vi "Console with Filter.vi"() -> ()   [LabVIEW 2019]
uses:
  Log/Log.lvclass
  Log Sinks/Sink-Console/Sink-Console.lvclass
  Log/Event Level.ctl
  TSC Event Logger.lvlib
  Layouts/SimpleLayout/SimpleLayout.lvclass
  Layouts/CSVLayout/CSVLayout.lvclass
  Layouts/JSONLayout/JSONLayout.lvclass
  Log Sinks/Sink-Console/Construct - Input.vi
  e05bdbe4-a397-4cd1-a311-50e4536787bd.vi
  C:/Development/Reuse-libraries/Event Logger/Layouts/Layout.lvclass
  C:/Development/Reuse-libraries/Event Logger/Log Sinks/Log Sinks.lvclass
panel:
  out "string array":string[][](array[string])
  in  "Level Filter":T1=enum."INFO"
  in  "Event Filter":string
  in  "Source Filter":string
  in  "Layout":enum16{"Simple", "CSV", "JSON"}(ring)
  out "String":string
  in  "Level":T1=enum."INFO"
  in  "Record Event":bool
  in  "Event Data":string="test"
  out "Error Out":errorcluster
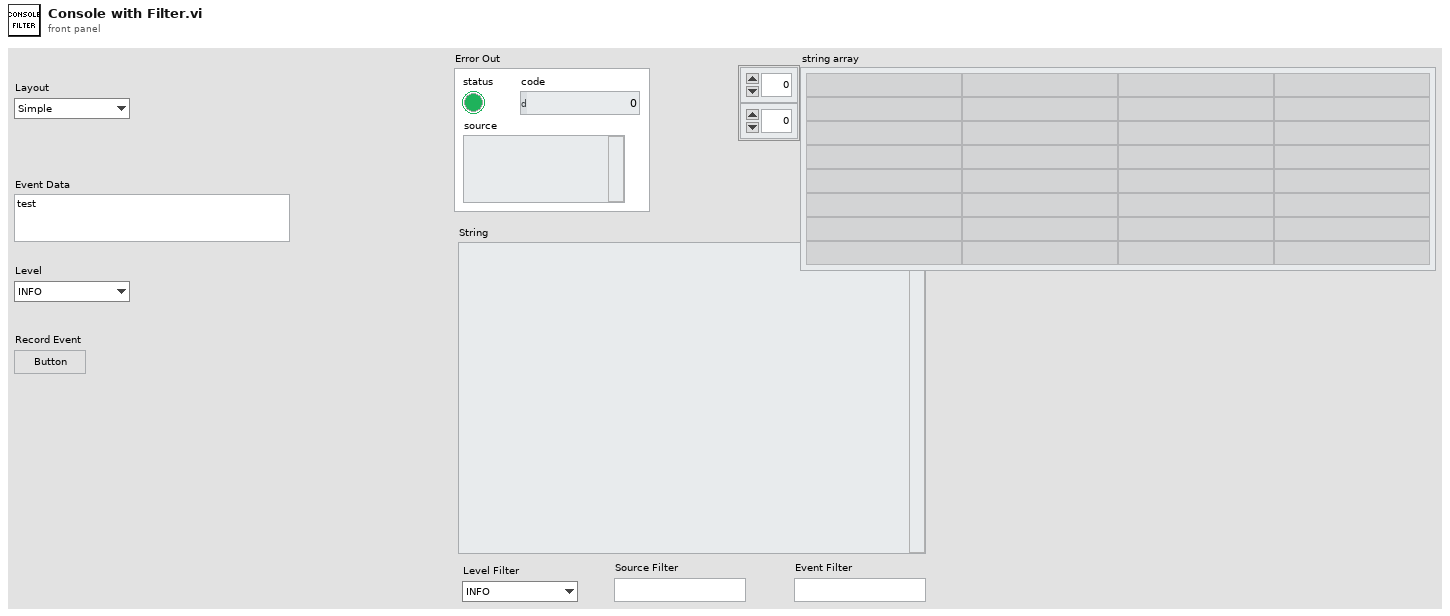
[diagram p1: front panel]
types:
  T1 = typedef "TSC Event Logger.lvlib/Event Level.ctl" = enum16{"OFF", "TRACE", "DEBUG", "INFO", "WARN", "ERROR", "FATAL"}
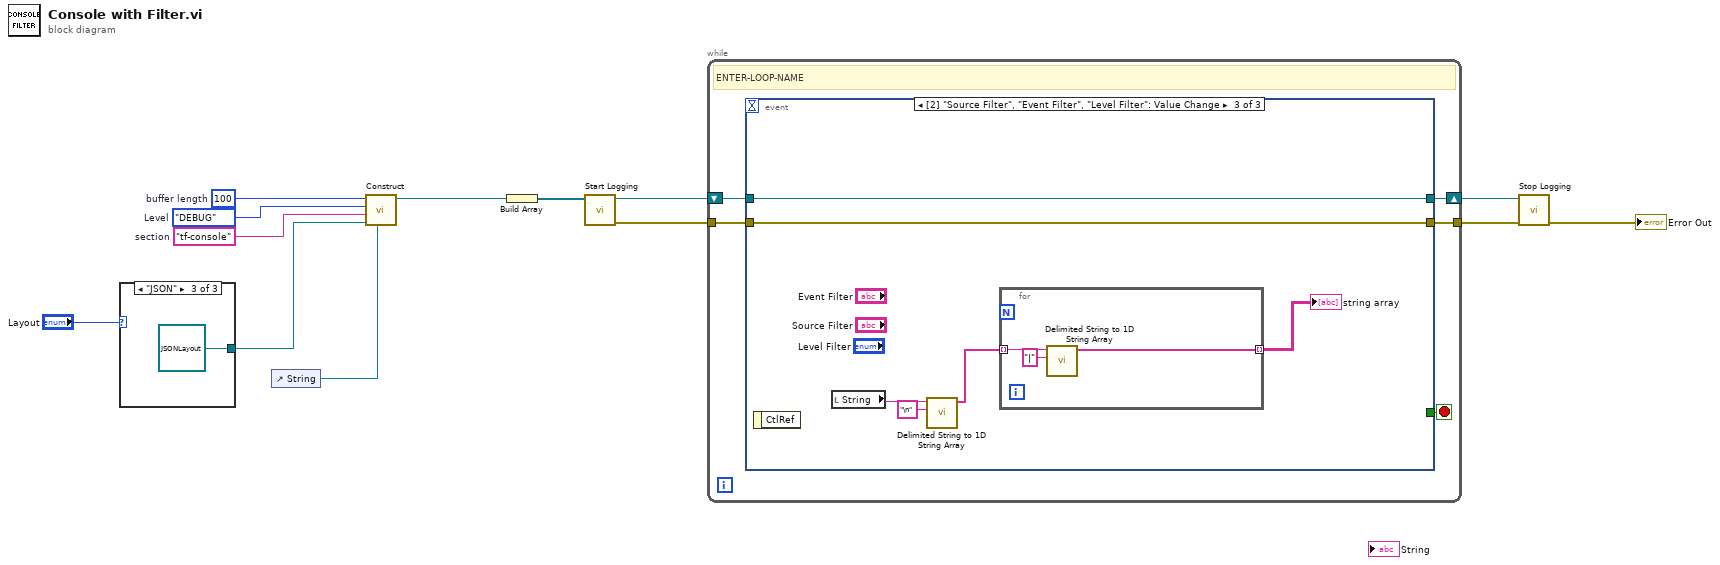
[diagram p0: block diagram]
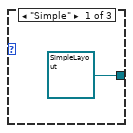
[diagram p2: hidden frame]
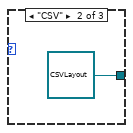
[diagram p3: hidden frame]
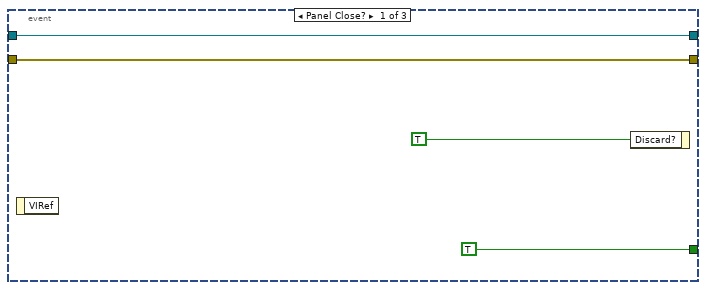
[diagram p4: hidden frame]
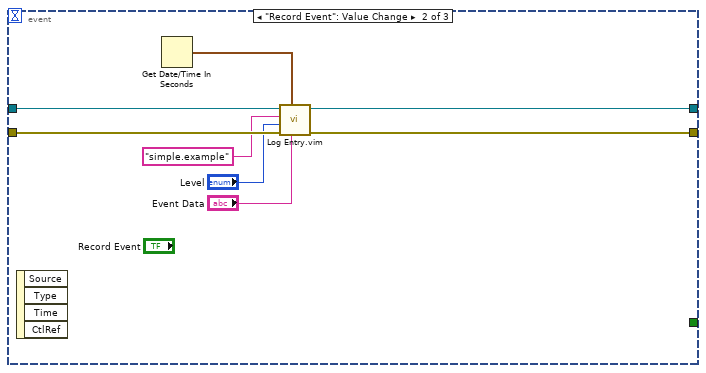
[diagram p5: hidden frame]
diagram:
  w3 = 100  # buffer length
  w4 = Event_Level."DEBUG"  # Level
  w5 = "tf-console"  # section
  n1 = case shown="\"JSON\"" "Layout" {
    tunnel: [refnum<class "SimpleLayout.lvclass"> refnum ("TSC Event Logger.lvlib:SimpleLayout.lvclass") refnum<class "CSVLayout.lvclass"> refnum ("TSC Event Logger.lvlib:CSVLayout.lvclass") refnum<class "JSONLayout.lvclass"> refnum ("TSC Event Logger.lvlib:JSONLayout.lvclass")] -> w1
    frame "Simple" {
    }
    frame "CSV" {
    }
    frame "JSON" {
    }
  }
  n2 = control-ref of="String"() -> (w6:refnum<vi>)
  n3 = call-poly "Construct.vi"("Console Ref"=w6, "Layout Type"=w1, "Name"=w5, "Level"=w4, "buffer length"=w3) -> ("Sink-Console"=w7:refnum<class "Sink-Console.lvclass">)  [unwired: 5 in, 1 out]
  n4 = Build Array(w7) -> (w8:refnum<class "Sink-Console.lvclass">[])
  n5 = call "Start Logging.vi"("Sinks"=w8) -> ("Error Out"=w12:errorcluster, "Logger"=w9:refnum<class "Log.lvclass">)  [unwired: 9 in]
  n6 = while {
    tunnel: w12 -> [w20]
    shift-right: [w18] -> w11
    shift-left: w9 -> [w19]
    tunnel: [w17] -> w10
    stop <- w21 stop-if-true
    # "ENTER-LOOP-NAME"
    n7 = event shown="[2] \"Source Filter\", \"Event Filter\", \"Level Filter\": Value Change" {
      selector: _ -> [_ _ _]
      dyn-events: _ -> [_ _ _]
      timeout: _ -> [_ _ _]
      tunnel: [TRUE _ _] -> w21
      tunnel: w20 -> [w22 w31 w38]
      tunnel: w19 -> [w23 w33 w39]
      tunnel: [w23 w32 w39] -> w18
      tunnel: [w22 w30 w38] -> w17
      event Panel Close? {
        n8 = event-data() -> ()  [unwired: 1 in, 1 out]
        n9 = event-data("Discard?"=TRUE) -> ()  [unwired: 1 in, 1 out]
      }
      event "Record Event": Value Change {
        n10 = event-data() -> ()  [unwired: 1 in, 4 out]
        n11 = Get Date/Time In Seconds() -> (seconds since 1Jan1904=w28:timestamp)
        n12 = call "Log Entry.vim"("Message"="Event Data", "Time"=w28, "error in (no error)"=w31, "Level"="Level", "Logger"="simple.example", "Log in"=w33) -> ("error out"=w30:errorcluster, "Log out"=w32:refnum<class "Log.lvclass">)  [unwired: 4 in]
      }
      event "Source Filter", "Event Filter": Value Change {
        n13 = event-data() -> ()  [unwired: 1 in, 1 out]
        n14 = local read "String"() -> (w37:string)
        n15 = call <vilib>:"Delimited String to 1D String Array.vi"("delimiter"="\n", "delimited string"=w37) -> ("string array"=w35:string[])  [unwired: 9 in]
        n16 = for {
          tunnel: w35 -> [w42] mode=indexing
          tunnel: [w40] -> w34 mode=indexing
          n17 = call <vilib>:"Delimited String to 1D String Array.vi"("delimiter"="|", "delimited string"=w42) -> ("string array"=w40:string[])  [unwired: 9 in]
        }
        "string array" <- w34
      }
    }
  }
  n18 = call "Stop Logging.vi"("Error In"=w10, "Logger"=w11) -> ("Error Out"=→"Error Out":errorcluster)  [unwired: 8 in, 1 out]
